vi "GetElementNames.vi"(8 "error in (no error)":errorcluster, 11 "ArrayElementScripter in":refnum<class "ArrayElementScripter.lvclass">) -> (0 "error out":errorcluster, 2 "Element Names":string[](array[string]), 3 "ArrayElementScripter out":refnum<class "ArrayElementScripter.lvclass">)   [LabVIEW 2021, in "MemberVICreation.lvlib" / "ArrayElementScripter.lvclass"]
uses:
  <resource>/Framework/Providers/LVClassLibrary/NewAccessors/ArrayElementScripter/ArrayElementScripter.lvclass
  <resource>/Framework/Providers/LVClassLibrary/NewAccessors/MemberVICreation.lvlib
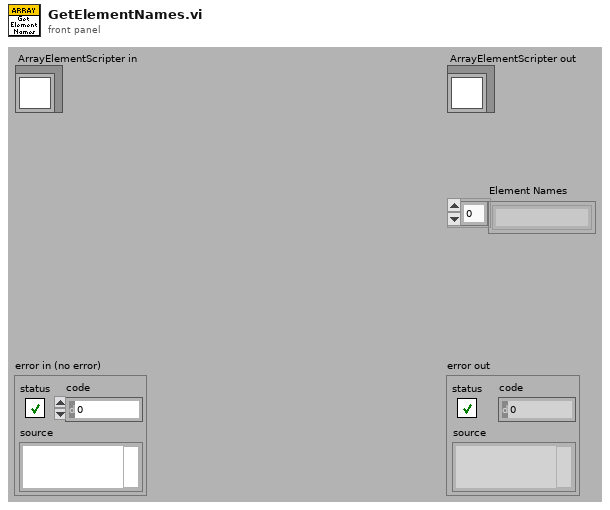
[diagram p1: front panel]
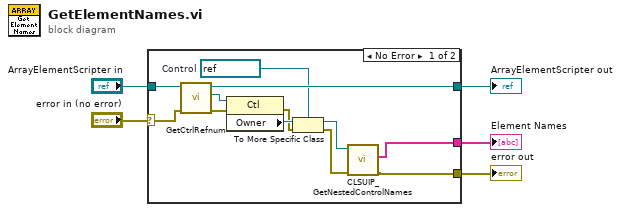
[diagram p0: block diagram]
diagram:
  n1 = case shown="No Error" "error in (no error)" {
    selector: "error in (no error)" -> [w16 w19]
    tunnel: [w7 w19] -> w4
    tunnel: "ArrayElementScripter in" -> [w17 w18]
    tunnel: [w6 _] -> w2
    tunnel: [w15 w18] -> w1
    frame No Error {
      w10 = refnum<vi> refnum  # Control
      n2 = call-dynamic "GetCtrlRefnum.vi"("error in (no error)"=w16, "BaseAccessorScripter in"=w17) -> ("error out"=w14:errorcluster, "Ctl Refnum"=w13:refnum<vi>, "BaseAccessorScripter out"=w15:refnum<class "ArrayElementScripter.lvclass">)  [unwired: 7 out]
      n3 = property class="Ctl"(reference=w13, error in=w14) -> (error out=w11:errorcluster, "Owner"=w12:refnum<vi>)  [unwired: 1 out]
      n4 = To More Specific Class(target class=w10, reference=w12, error in=w11) -> (specific class reference=w9:refnum<vi>, error out=w8:errorcluster)
      n5 = call <resource>:"CLSUIP_GetNestedControlNames.vi"("error in (no error)"=w8, "Ctl Refnum"=w9) -> ("error out"=w7:errorcluster, "Element names"=w6:string[])  [unwired: 8 out]
    }
    frame Error {
    }
  }
  "error out" <- w4
  "Element Names" <- w2
  "ArrayElementScripter out" <- w1
